vi "Solve1.vi"(8 "Error In":errorcluster, 11 "object in":refnum<class "2024_5.lvclass">) -> (0 "Error Out":errorcluster, 2 "Result":u64, 3 "object out":refnum<class "2024_5.lvclass">)   [LabVIEW 2023, in "2024_5.lvclass"]
uses:
  2024_5.lvclass
  2024_5.lvclass/2024_5.ctl
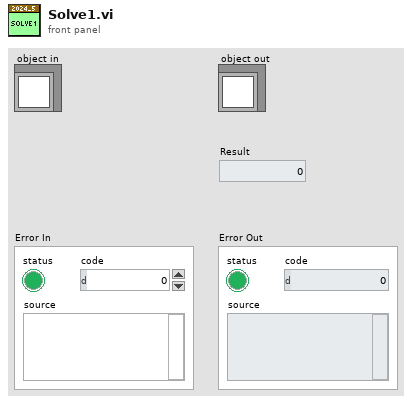
[diagram p1: front panel]
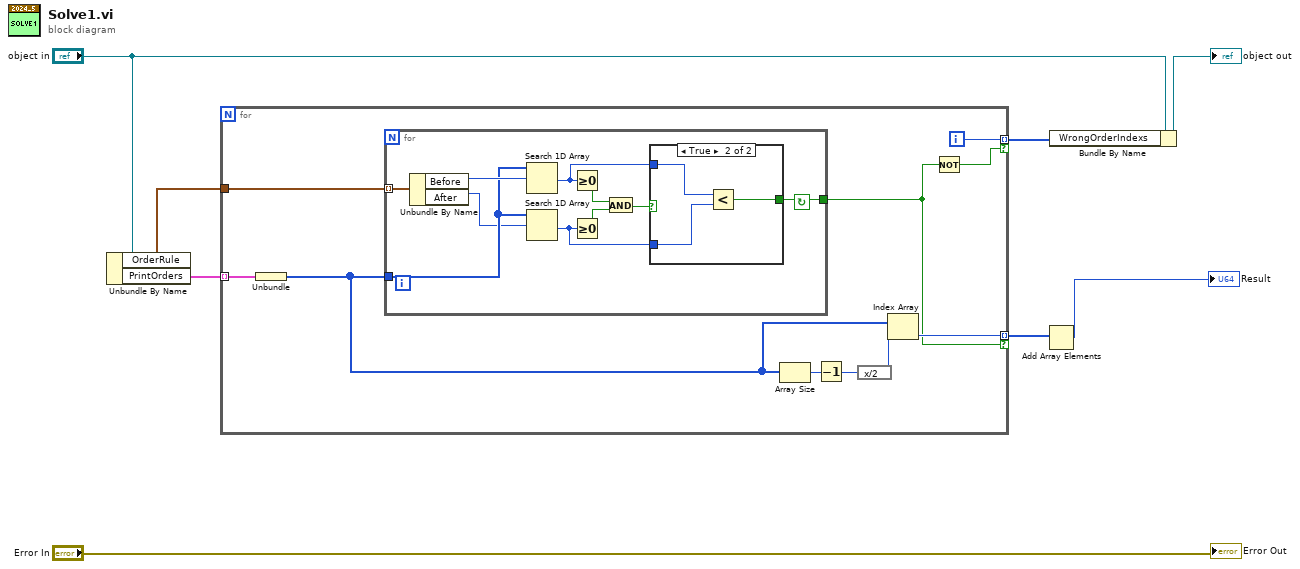
[diagram p0: block diagram]
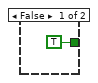
[diagram p2: hidden frame]
diagram:
  n1 = Unbundle By Name("object in") -> ("OrderRule"=w5:cluster{"Before":i64, "After":i64}[], "PrintOrders"=w6:cluster{"Pages":i32[]}[])
  n2 = for {
    tunnel: w6 -> [w18] mode=indexing
    tunnel: w5 -> [w17]
    tunnel: [w12] -> w4 mode=indexing if=w11
    tunnel: [w10] -> w1 mode=indexing if=w9
    i -> [w10]
    n3 = Unbundle(w18) -> ("Pages"=w14:i32[])
    n4 = for {
      tunnel: w17 -> [w28] mode=indexing
      tunnel: w14 -> [w26]
      tunnel: [w19] -> w11
      stop <- w19 continue-if-true
      n5 = Unbundle By Name(w28) -> ("Before"=w27:i64, "After"=w25:i64)
      n6 = Search 1D Array(1D array=w26, element=w27) -> (index of element=w21:i32)  [unwired: 1 in]
      n7 = Search 1D Array(1D array=w26, element=w25) -> (index of element=w20:i32)  [unwired: 1 in]
      n8 = Greater Or Equal To 0?(x=w21) -> (x >= 0?=w23:bool)
      n9 = Greater Or Equal To 0?(x=w20) -> (x >= 0?=w24:bool)
      n10 = And(x=w23, y=w24) -> (x .and. y?=w22:bool)
      n11 = case shown="True" w22 {
        tunnel: w21 -> [_ w32]
        tunnel: w20 -> [_ w31]
        tunnel: [TRUE w30] -> w19
        frame False {
        }
        frame True {
          n12 = Less?(x=w32, y=w31) -> (x < y?=w30:bool)
        }
      }
    }
    n13 = Array Size(array=w14) -> (size(s)=w16:i32)
    n14 = Decrement(x=w16) -> (x-1=w15:i32)
    n15 = expression code="x/2"(w15) -> (w13:i32)
    n16 = Index Array(array=w14, index=w13) -> (element=w12:i32)
    n17 = Not(x=w11) -> (.not. x?=w9:bool)
  }
  n18 = Add Array Elements(numeric array=w4) -> (sum=→"Result":i32)
  n19 = Bundle By Name(cluster="object in", "WrongOrderIndexs"=w1) -> (→"object out":refnum<class "2024_5.lvclass">)
  "Error Out" <- "Error In"
